vi "MPC-200 Wrapper for U command.vi"(8 "error in (no error)":errorcluster, 11 "VISA resource name in":refnum<visa-resource-name>) -> (0 "error out":errorcluster, 1 "Connector statuses":u8[](array[numeric]), 2 "num controllers connected":u8, 3 "VISA resource name out":refnum<visa-resource-name>)   [LabVIEW 2015, in "XYZStage.lvlib"]
uses:
  XYZStage.lvlib
  <vilib>/Utility/error.llb/Error Cluster From Error Code.vi
  <vilib>/ErrorRing/Error Ring.xnode
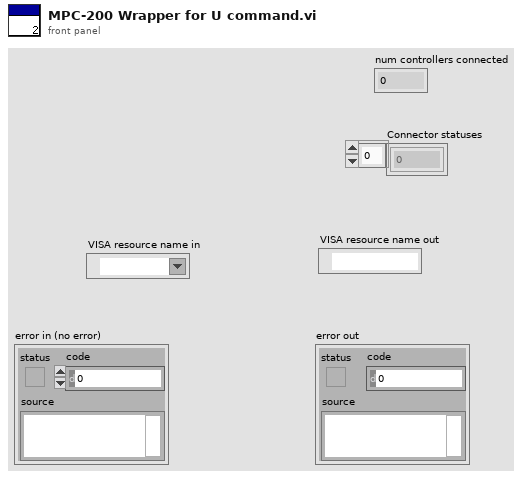
[diagram p1: front panel]
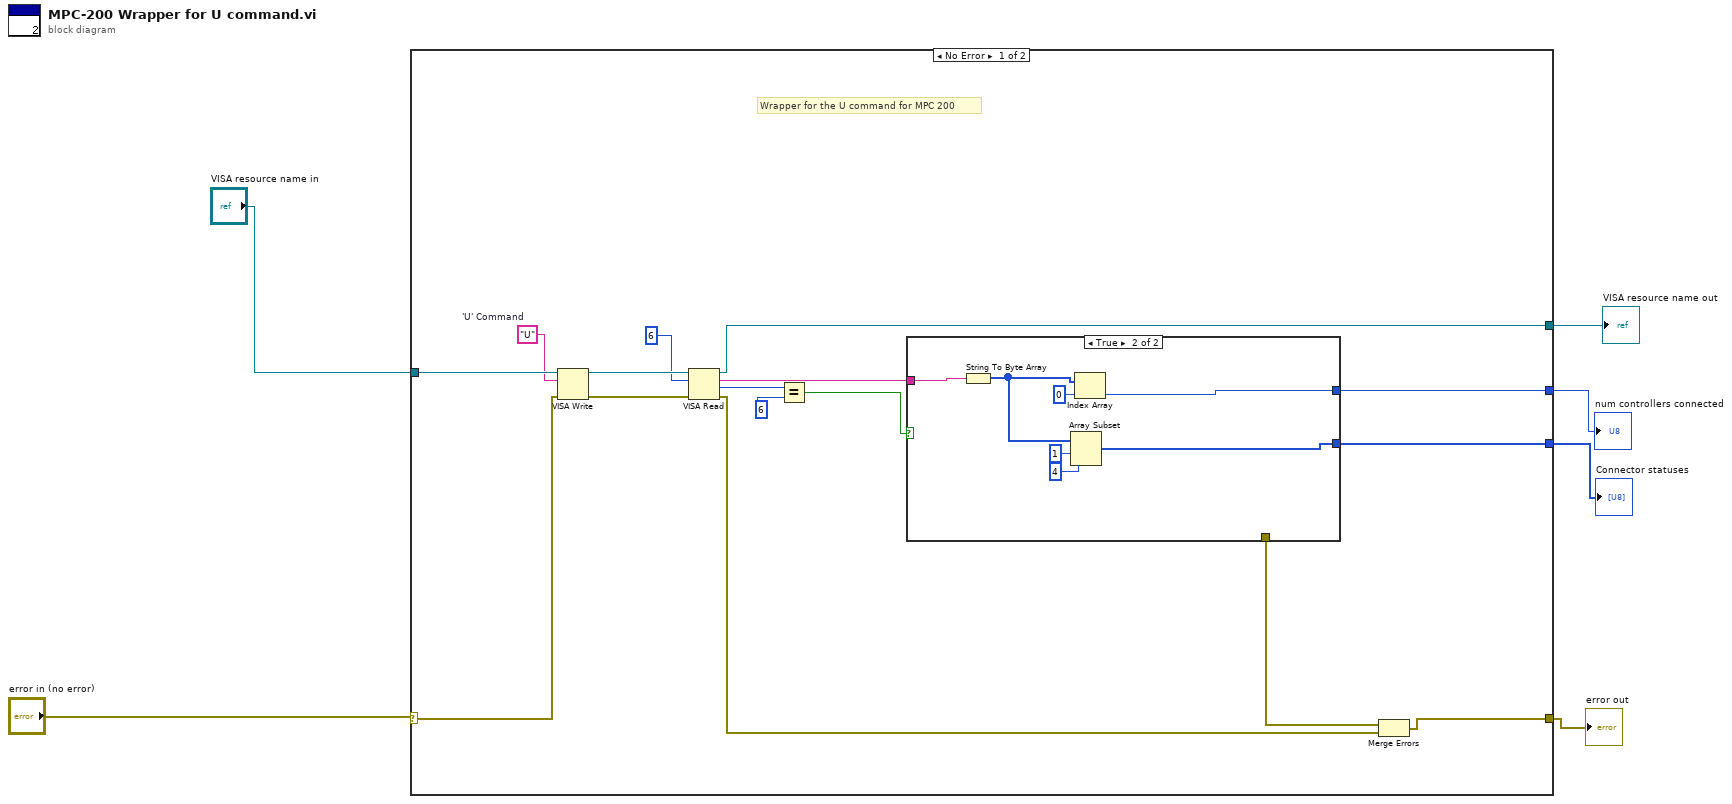
[diagram p0: block diagram]
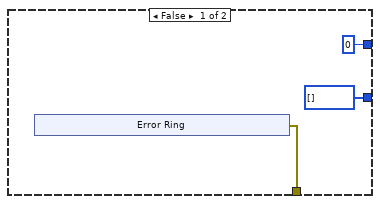
[diagram p2: hidden frame]
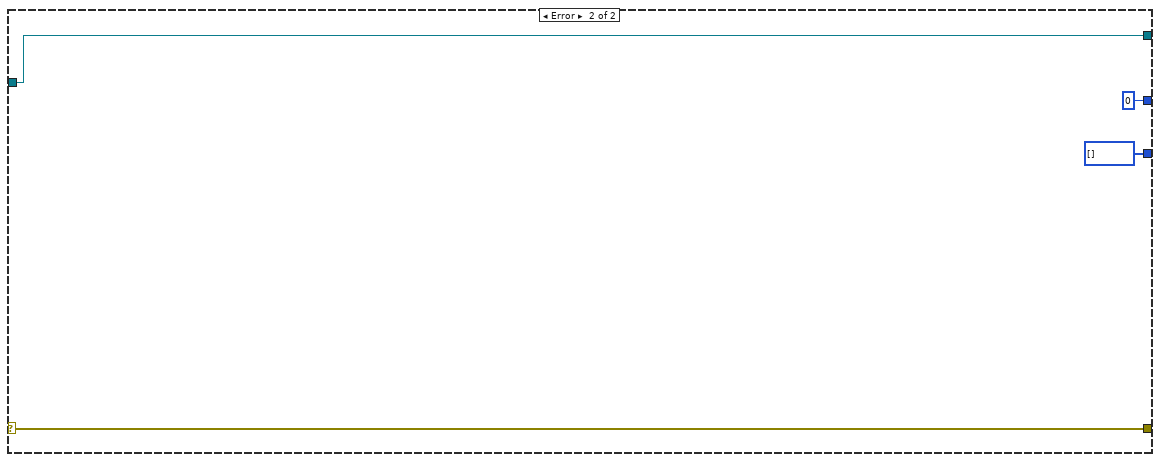
[diagram p3: hidden frame]
diagram:
  n1 = case shown="No Error" "error in (no error)" {
    selector: "error in (no error)" -> [w21 w41]
    tunnel: [w9 w41] -> w5
    tunnel: "VISA resource name in" -> [w22 w40]
    tunnel: [w16 w40] -> w3
    tunnel: [w14 u8 0] -> w2
    tunnel: [w13 u8[] []] -> w1
    frame No Error {
      w19 = "U"  # 'U' Command
      # "Wrapper for the U command for MPC 200"
      n2 = VISA Write(VISA resource name=w22, write buffer=w19, error in (no error)=w21) -> (VISA resource name out=w18:refnum<visa-resource-name>, error out=w20:errorcluster)  [unwired: 1 out]
      n3 = VISA Read(VISA resource name=w18, byte count=u32 6, error in (no error)=w20) -> (VISA resource name out=w16:refnum<visa-resource-name>, read buffer=w15:string, return count=w12:u32, error out=w7:errorcluster)
      n4 = Equal?(x=w12, y=u32 6) -> (x = y?=w10:bool)
      n5 = case shown="True" w10 {
        tunnel: w15 -> [_ w37]
        tunnel: [u8 0 w35] -> w14
        tunnel: [u8[] [] w31] -> w13
        tunnel: [w25 _] -> w8
        frame False {
          n6 = xnode "Error Ring"() -> ("error out"=w25:errorcluster)
        }
        frame True {
          n7 = String To Byte Array(string=w37) -> (unsigned byte array=w34:u8[])
          n8 = Array Subset(array=w34, index=1, length=4) -> (w31:u8[])
          n9 = Index Array(array=w34, index=0) -> (element=w35:u8)
        }
      }
      n10 = Merge Errors(w8, w7) -> (w9:errorcluster)
    }
    frame Error {
    }
  }
  "VISA resource name out" <- w3
  "error out" <- w5
  "num controllers connected" <- w2
  "Connector statuses" <- w1
